vi "Configure Marker.vi"(0 "VISA resource name":refnum<visa-resource-name>, 5 "Marker Mode (0: Off)":i32(ring) items=["Off", "Position", "RMS (Degree)", "RMS (Radian)", "RFM", "RMS (Jitter)"], 7 "Select Marker (1: Marker 1)":i32(ring)=1 items=["Marker 1"=1, "Marker 2"=2, "Marker 3"=3, "Marker 4"=4], 9 "Select Marker Trace (1: Trace 1)":i32(ring)=1 items=["Trace 1"=1, "Trace 2"=2, "Trace 3"=3], 11 "error in (no error)":errorcluster, 12 "Marker X-Axis Position (10 kHz)":dbl=10000.0) -> (4 "VISA resource name out":refnum<visa-resource-name>, 15 "error out":errorcluster)   [LabVIEW 2014, in "Agilent ESA PSA Series.lvlib"]
doc: "Configures the markers for the Log Plot measurement of the Phase Noise personality. Call this VI twice for the marker functions <B>RMS (Radian), RMS (Degrees), RFM, RMS (Jitter)</B> which require a period. Both calls should have the same settings except <B>Marker X-Axis Position</B>.\n\n<B>Note:</B> \n\nThis VI is only valid in Phase Noise personality. Use <B>Switch Personality</B> VI to switch to Phase Noise before calling this VI."
uses:
  Agilent ESA PSA Series.lvlib
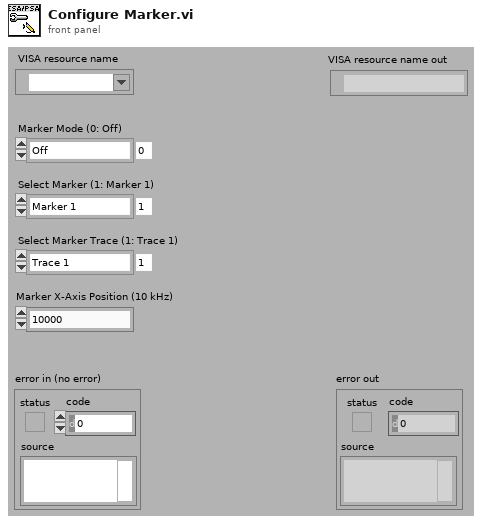
[diagram p1: front panel]
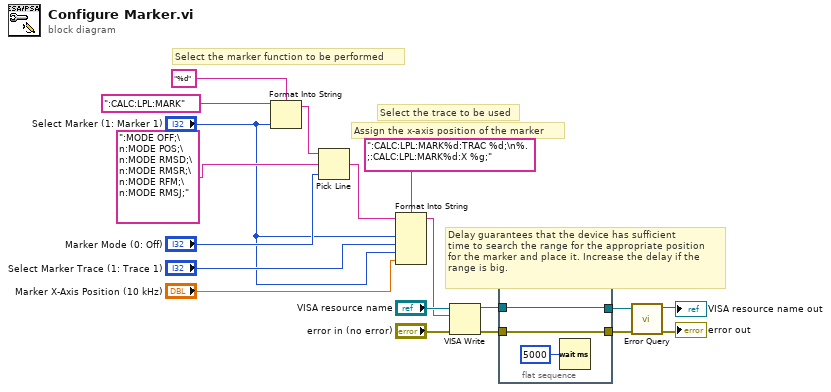
[diagram p0: block diagram]
diagram:
  # "Delay guarantees that the device has sufficient\ntime to search the range for the appropriate position\nfor the marker and place it. Increase the delay if the\nrange is big."
  # "Assign the x-axis position of the marker"
  # "Select the trace to be used"
  # "Select the marker function to be performed"
  n1 = Format Into String(format string="%d", initial string=":CALC:LPL:MARK", "Select Marker (1: Marker 1)") -> (resulting string=w11:string)  [unwired: 1 in, 1 out]
  n2 = Pick Line(string ("")=w11, multi-line string=":MODE OFF;\n:MODE POS;\n:MODE RMSD;\n:MODE RMSR;\n:MODE RFM;\n:MODE RMSJ;", line index="Marker Mode (0: Off)") -> (output string=w10:string)
  n3 = Format Into String(format string=":CALC:LPL:MARK%d:TRAC %d;\n%.;:CALC:LPL:MARK%d:X %g;", initial string=w10, "Select Marker (1: Marker 1)", "Select Marker Trace (1: Trace 1)", "Select Marker (1: Marker 1)", "Marker X-Axis Position (10 kHz)") -> (resulting string=w5:string)  [unwired: 1 in, 1 out]
  n4 = VISA Write(VISA resource name="VISA resource name", write buffer=w5, error in (no error)="error in (no error)") -> (VISA resource name out=w4:refnum<visa-resource-name>, error out=w3:errorcluster)  [unwired: 1 out]
  n5 = flat-sequence {
    tunnel: w4 -> [w22]
    tunnel: w3 -> [w21]
    tunnel: [w22] -> w2
    tunnel: [w21] -> w1
    frame #0 {
      n6 = Wait (ms)(milliseconds to wait=u32 5000) -> ()  [unwired: 1 out]
    }
  }
  n7 = call "Error Query.vi"("error in (no error)"=w1, "VISA resource name"=w2) -> ("error out"=→"error out":errorcluster, "VISA resource name out"=→"VISA resource name out":refnum<visa-resource-name>)  [unwired: 6 in, 2 out]
